vi "Write Port.vi"(0 "Serial Device in":refnum<class "Serial Device.lvclass">, 5 "VISA resource name":refnum<visa-resource-name>, 7 "Binary Number":T1, 9 "Port 2":dbl, 11 "error in (no error)":errorcluster) -> (4 "Serial Device out":refnum<class "Serial Device.lvclass">, 8 "VISA resource name 2":refnum<visa-resource-name>, 10 "Response":string, 15 "error out":errorcluster)   [LabVIEW 2020, in "Serial Device.lvclass"]
uses:
  Serial Device.lvclass
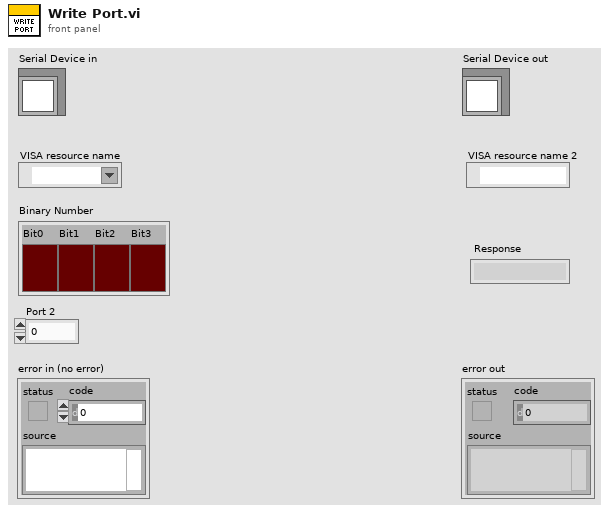
[diagram p1: front panel]
types:
  T1 = cluster{"Bit0":bool, "Bit1":bool, "Bit2":bool, "Bit3":bool}
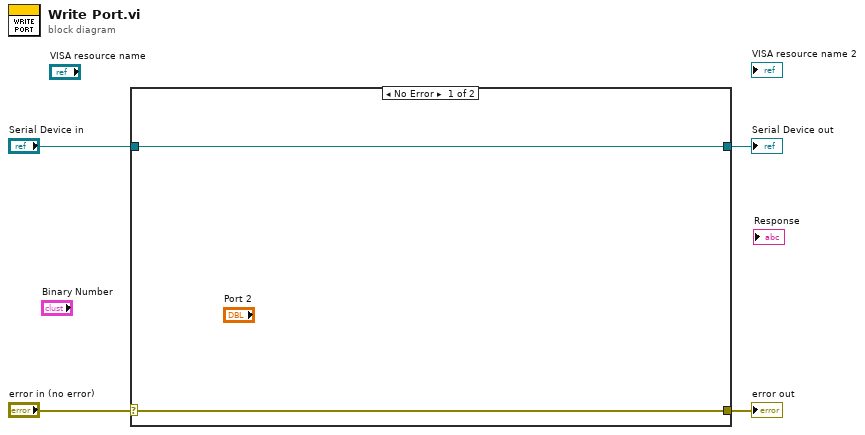
[diagram p0: block diagram]
diagram:
  n1 = case shown="No Error" "error in (no error)" {
    selector: "error in (no error)" -> [w5 w8]
    tunnel: [w5 w8] -> w3
    tunnel: [w6 w7] -> w1
    tunnel: "Serial Device in" -> [w6 w7]
    frame No Error {
    }
    frame Error {
    }
  }
  "error out" <- w3
  "Serial Device out" <- w1
